vi "手动控制.vi"() -> ()   [LabVIEW 2016]
uses:
  Controls/robotdata.ctl
  <vilib>/Utility/miscctls.llb/LVRGBAColorTypeDef.ctl
  <vilib>/LabVIEW Interface for Arduino/LabVIEW Interface for Arduino.lvlib
panel:
  in  "背景色":u32(colorbox)=15204350
  in  "转    台：":sgl(slide) scale=0.0..90.0 scale format="%#_g°"
  in  "手    臂：":sgl(slide) scale=0.0..90.0 scale format="%#_g°"
  in  "上下移动：":dbl(slide)=6.46551724137931 scale=0.0..100.0
  in  "拇指":sgl(slide) caption="拇    指：" scale=0.0..60.0 scale format="%#_g°"
  in  "食    指：":sgl(slide) caption="食指" scale=0.0..90.0 scale format="%#_g°"
  in  "中    指：":sgl(slide) caption="中指" scale=0.0..90.0 scale format="%#_g°"
  in  "无名指：":sgl(slide) caption="无名指" scale=0.0..90.0 scale format="%#_g°"
  in  "小手指：":sgl(slide) caption="小手指" scale=0.0..90.0 scale format="%#_g°"
  in  "手    腕：":sgl(slide) scale=0.0..90.0 scale format="%#_g°"
  in  "hand":T1={"手腕"=52.38806, "小手指"=0.0, "无名指"=0.0, "中指"=0.0, "食指"=0.0, "上下移动"=-1.8918918918918917, "背景色"=15204350, "拇指"=0.0, "转台"=52.38806, "手臂"=52.38806} {"手臂" scale=0.0..90.0; "转台" scale=0.0..360.0; "拇指" scale=0.0..90.0; "上下移动" scale=0.0..100.0; "食指" scale=0.0..90.0; "中指" scale=0.0..90.0; "无名指" scale=0.0..90.0; "小手指" scale=0.0..90.0; "手腕" scale=0.0..360.0}
  out "机械手":refnum<vi>(3d-picture)
  in  "退出":bool=TRUE
  # "创世捷能 CSJN"
  # "趣味机械手"
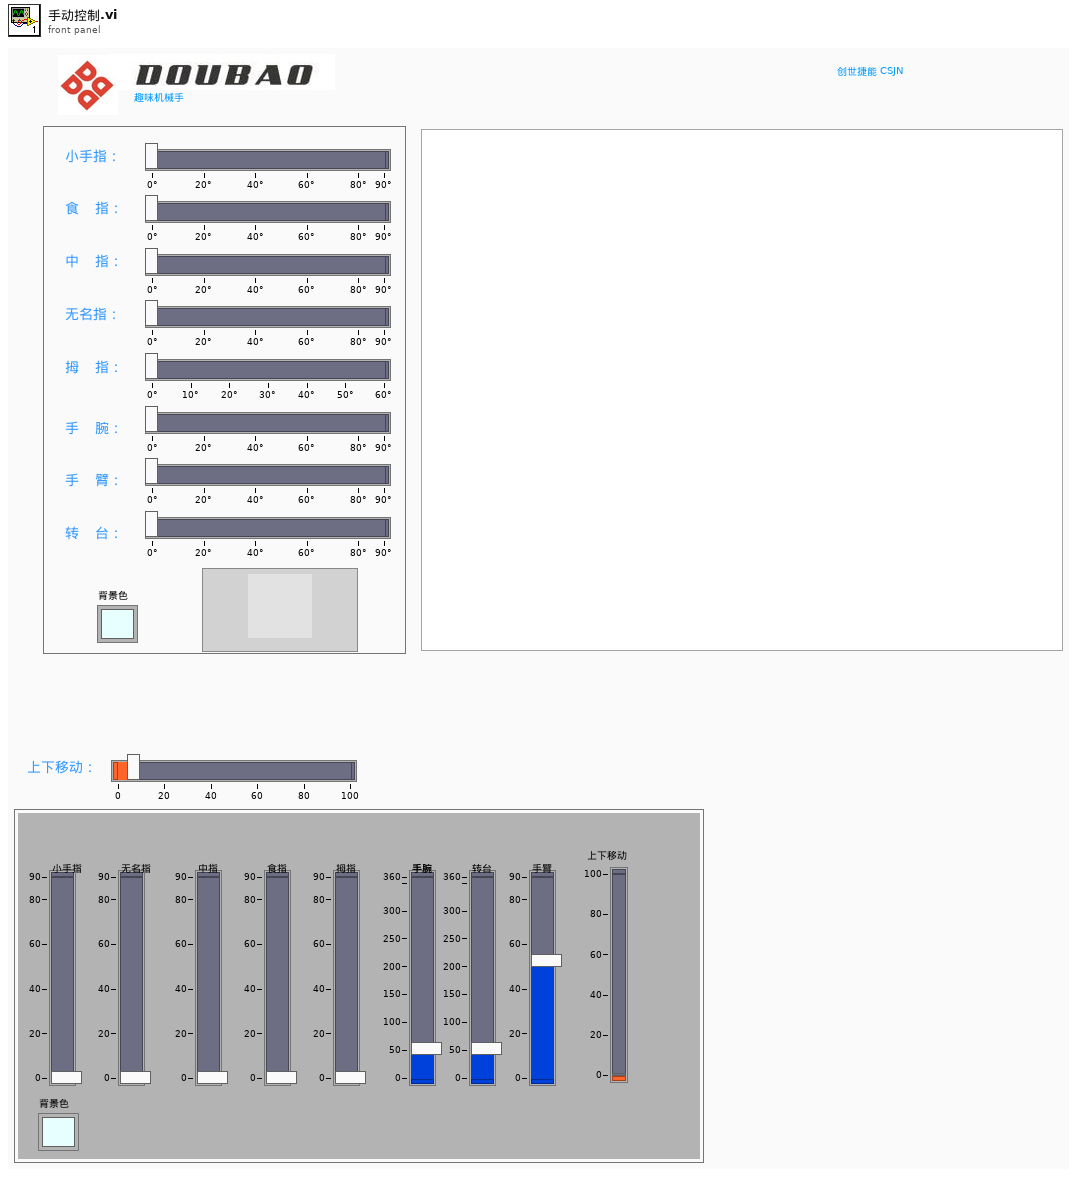
[diagram p1: front panel]
types:
  T1 = typedef "robotdata.ctl" = cluster{"手腕":sgl, "小手指":sgl, "无名指":sgl, "中指":sgl, "食指":sgl, "上下移动":dbl, "背景色":u32, "拇指":sgl, "转台":sgl, "手臂":sgl}
  T2 = typedef "LabVIEW Interface for Arduino.lvlib/Arduino Resource.ctl" = cluster{"VISA resource":refnum<visa-resource-name>, "Board Type":T3, "Connection Type":enum8{"USB / Serial"}, "Bytes Per Packet (15)":u8}
  T3 = typedef "LabVIEW Interface for Arduino.lvlib/Board Type.ctl" = enum16{"Uno", "Dimuelanove w/Atmega 328", "Mega 2560"}
  T4 = typedef "handdata.ctl" = cluster{"机械手":refnum<vi>, "转台":refnum<vi>, "手臂":refnum<vi>, "手腕":refnum<vi>, "拇指指尖":refnum<vi>, "拇指指中 ":refnum<vi>, "食指指中":refnum<vi>, "食指指尖":refnum<vi>, "中指指中":refnum<vi>, "中指指尖":refnum<vi>, "无名指指中":refnum<vi>, "无名指指尖":refnum<vi>, "小手指指中":refnum<vi>, "小手指指尖":refnum<vi>}
  T5 = typedef "LVRGBAColorTypeDef.ctl" = cluster{"Red":sgl, "Green":sgl, "Blue":sgl, "Alpha":sgl}
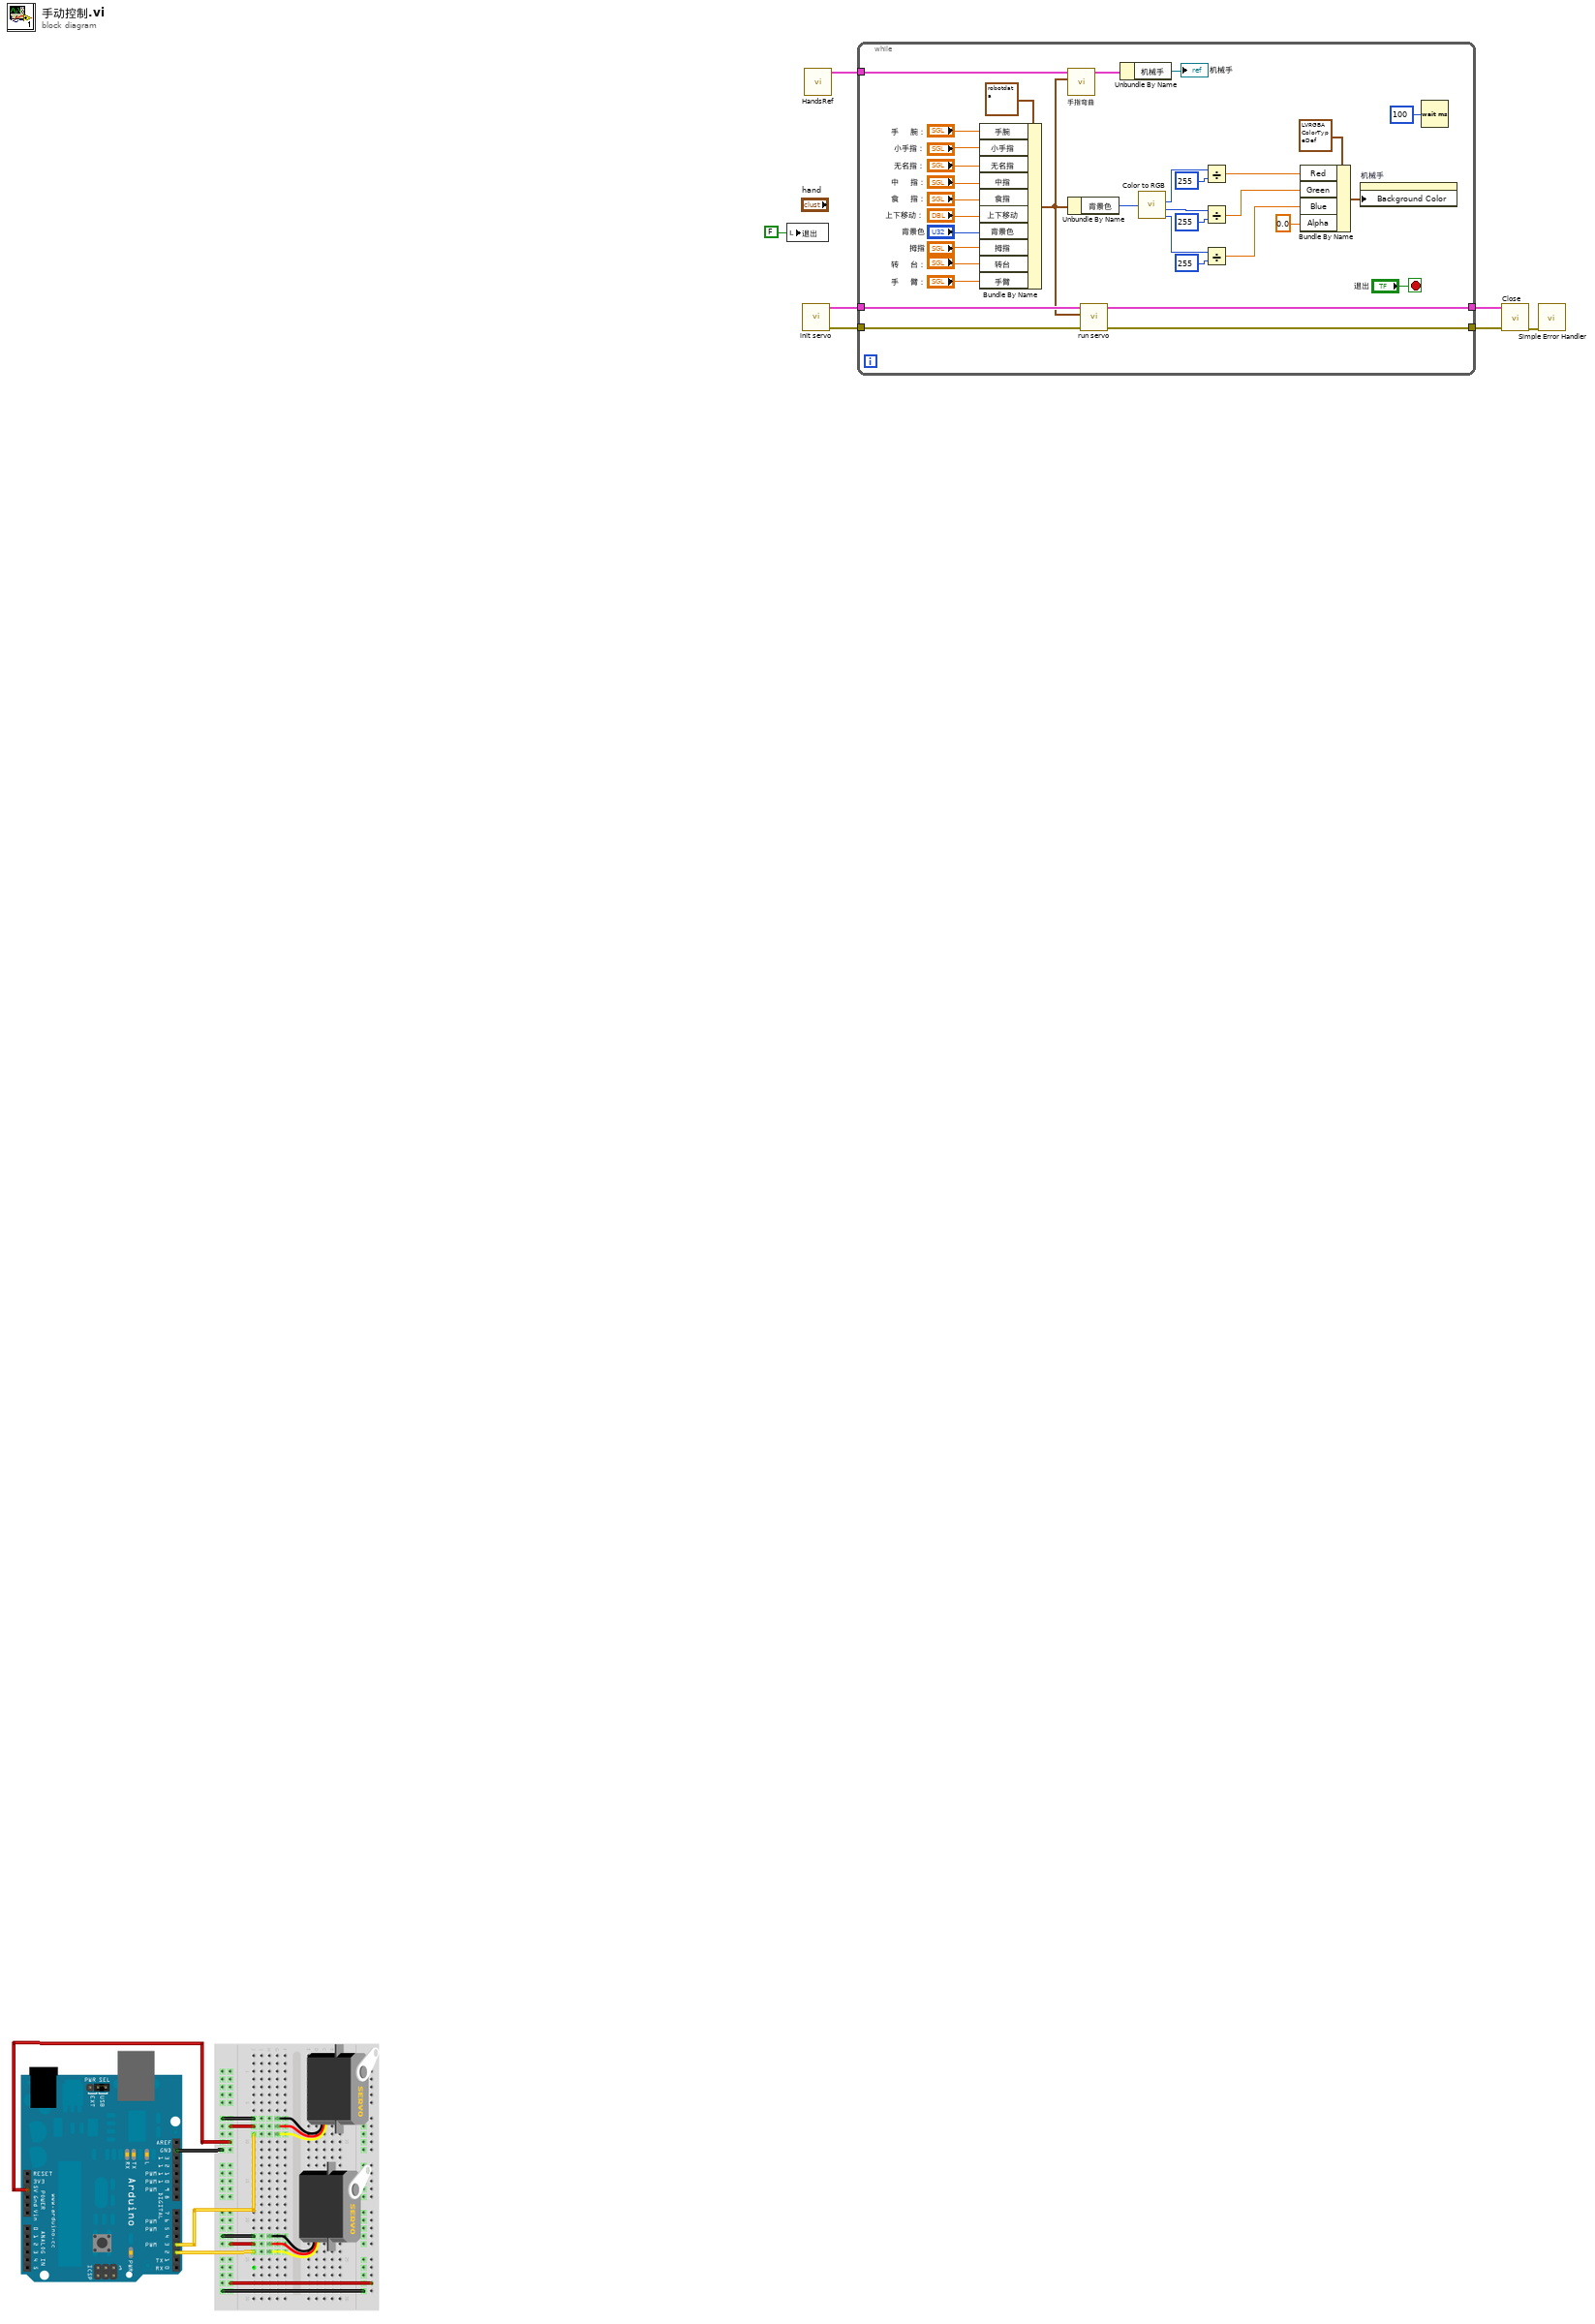
[diagram p0: block diagram]
diagram:
  n1 = local write "退出"(FALSE ("退出")) -> ()
  n2 = call "init servo.vi"() -> ("错误输出"=w3:errorcluster, "Arduino Resource"=w5:T2)  [unwired: 10 in]
  n3 = call "HandsRef.vi"() -> ("簇"=w6:T4)  [unwired: 9 in, 2 out]
  n4 = while {
    tunnel: w6 -> [w27]
    tunnel: w5 -> [w12]
    tunnel: [w11] -> w4
    tunnel: w3 -> [w10]
    tunnel: [w9] -> w2
    stop <- "退出" stop-if-true
    n5 = Bundle By Name(cluster=T1 {"手腕"=52.38806, "小手指"=0.0, "无名指"=0.0, "中指"=0.0, "食指"=0.0, "上下移动"=-1.8918918918918917, "背景色"=15204350, "拇指"=0.0, "转台"=52.38806, "手臂"=52.38806} ("hand"), "手腕"="手    腕：", "小手指"="小手指：", "无名指"="无名指：", "中指"="中    指：", "食指"="食    指：", "上下移动"="上下移动：", "背景色"="背景色", "拇指"="拇指", "转台"="转    台：", "手臂"="手    臂：") -> (w8:T1)
    n6 = call "手指弯曲.vi"("Hands Data In"=w8, "Hands Ref In"=w27) -> ("Hands Ref Out"=w26:T4)  [unwired: 7 in, 2 out]
    n7 = Unbundle By Name(w8) -> ("背景色"=w29:u32)
    n8 = call "run servo.vi"("错误输入（无错误）"=w10, "hand"=w8, "Arduino Resource输入"=w12) -> ("错误输出"=w9:errorcluster, "Arduino Resource输出"=w11:T2)  [unwired: 7 in]
    n9 = Unbundle By Name(w26) -> ("机械手"=→"机械手":refnum<vi>)
    n10 = call <vilib>:"Color to RGB.vi"("Color"=w29) -> ("R"=w33:u8, "G"=w34:u8, "B"=w30:u8)  [unwired: 1 out]
    n11 = Divide(x=w33, y=u32 255) -> (x/y=w38:dbl)
    n12 = Divide(x=w34, y=u32 255) -> (x/y=w35:dbl)
    n13 = Divide(x=w30, y=u32 255) -> (x/y=w31:dbl)
    n14 = Bundle By Name(cluster=T5 {"Red"=0.7, "Green"=0.7, "Blue"=0.7, "Alpha"=0.0} ("背景色"), "Red"=w38, "Green"=w35, "Blue"=w31, "Alpha"=sgl 0.0) -> (w41:T5)
    n15 = property on="机械手" class="SceneGraphDisp (严格)"("Background Color"=w41) -> ()  [unwired: 2 in, 2 out]
    n16 = Wait (ms)(milliseconds to wait=u32 100 ("等待时间（毫秒）")) -> ()  [unwired: 1 out]
  }
  n17 = call <vilib>:"Close.vi"("Arduino Resource"=w4, "error in"=w2) -> ("error out"=w1:errorcluster)  [unwired: 13 in]
  n18 = call <vilib>:"Simple Error Handler.vi"("error in (no error)"=w1) -> ()  [unwired: 4 in, 5 out]
